vi "Multiscale Pyramids.vi"() -> ()   [LabVIEW 2023]
uses:
  Images/_Images.ctl
  SubVIs/FLT/Conv Flt Presets.ctl
  <vilib>/vision/NI_Vision_Development_Module.lvlib
panel:
  out "Pyr Levels":i32=9
  in  "Filters":T1[](array[typedef])=[enum."Seifert 7x7", enum."Seifert 5x5", enum."Highlight Details 3x3", enum."None", enum."None", enum."None", enum."None", enum."None", enum."None", enum."None", enum."None", enum."None"]
  out "Histogram":T2(graph)
  in  "Operator":u16(ring)=6 items=["Linear", "Log", "Exp", "Square", "Square root", "Power X", "Power 1/X"]
  in  "X Value":sgl=1.2 format="%.2f"
  in  "Threshold":sgl=30.0
  in  "Radius":sgl=33.0
  in  "Amount":sgl=6.0
  in  "LUT Multiplier":sgl[](array[slide])=[157.53847, 185.1077, 192.98462, 248.12308, 196.92308, 248.12308, 252.06154, 114.215385, 248.12308, 110.276924, 102.4, 102.4] scale=0.0..512.0
  in  "LUT Power":sgl[](array[slide])=[0.61538464, 0.43076923, 0.3846154, 0.43846154, 0.42307693, 0.5538462, 0.64615387, 0.61538464, 0.61538464, 0.6, 0.4, 0.4] scale=0.0..2.0
  out "Reconstructed Image":T3(plugin-control)
  out "Source Image":T3(plugin-control)
  in  "Image":T4=enum."Part1"
  # "Multoscale Contrast Enhancement using Pyramids"
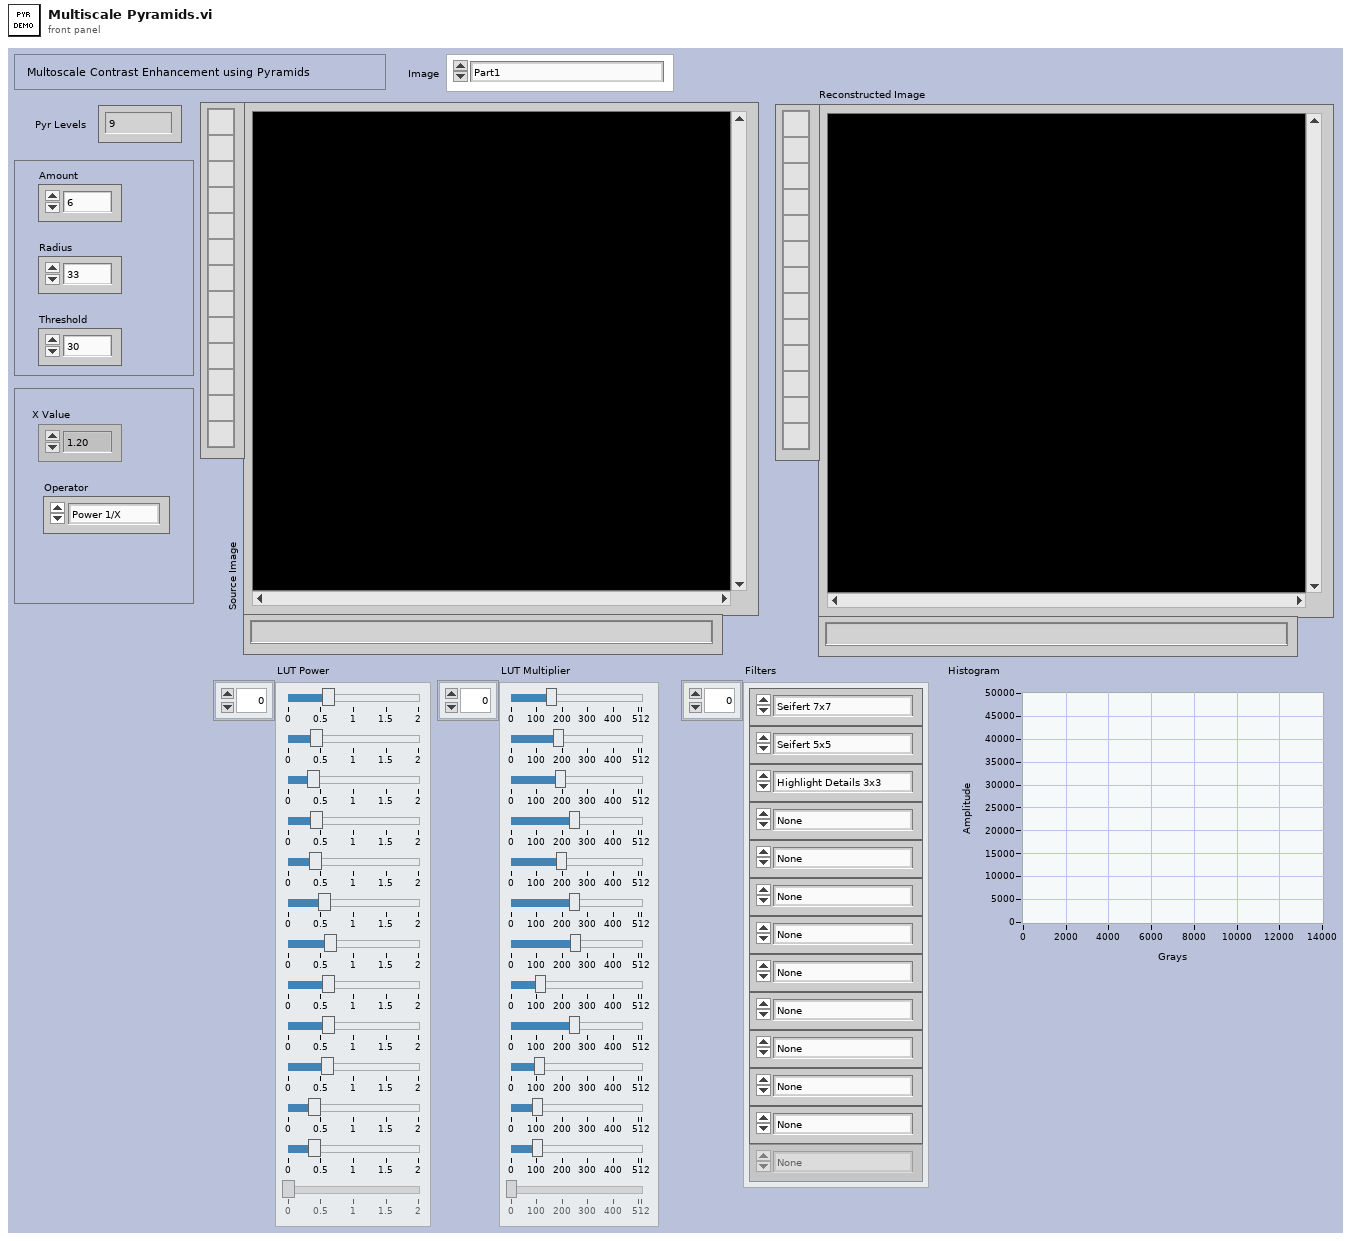
[diagram p1: front panel]
types:
  T1 = typedef "Conv Flt Presets.ctl" = enum16{"None", "Seifert 5x5", "Seifert 7x7", "High Pass 5x5 ", "High Pass 7x7", "Highlight Details 3x3", "Highlight Details 5x5", "Highlight Detail 7x7"}
  T2 = cluster{"Starting Value":sgl, "Incremental Value":sgl, "Histogram":u32[]}
  T3 = typedef "IMAQ Image.ctl" = refnum<image>
  T4 = typedef "_Images.ctl" = enum16{"Balls2", "Battery1", "Battery2", "Connector1", "Subwoofer1", "Subwoofer2", "Subwoofer3", "Subwoofer4", "Hase1", "Lamp1", "Lamp2", "Mouse1", "PhotoLens1", "Po1", "PowerSupply1", "Router", "--- Step Wedges ---", "Stepwedge1", "Stepwedge2", "Stepwedge3", "--- Fusion ---", "Fusion160kV", "Fusion2-120kV", "Fusion2-320kV", "Fusion300kV", "FusionPart1-120kV", "FusionPart1-180kV", "--- PART 01 ---", "Part1", "Part2", "Part3", "Part4", "Part5", "Part6", "Part7", "Part8", "--- Different Integrations ---", "Step2737-02Int", "Step2737-04Int", "Step2737-08Int", "Step2737-16Int", "Step2737-32Int", "Step2737-64Int"}
  T5 = typedef "Image Type" = u32
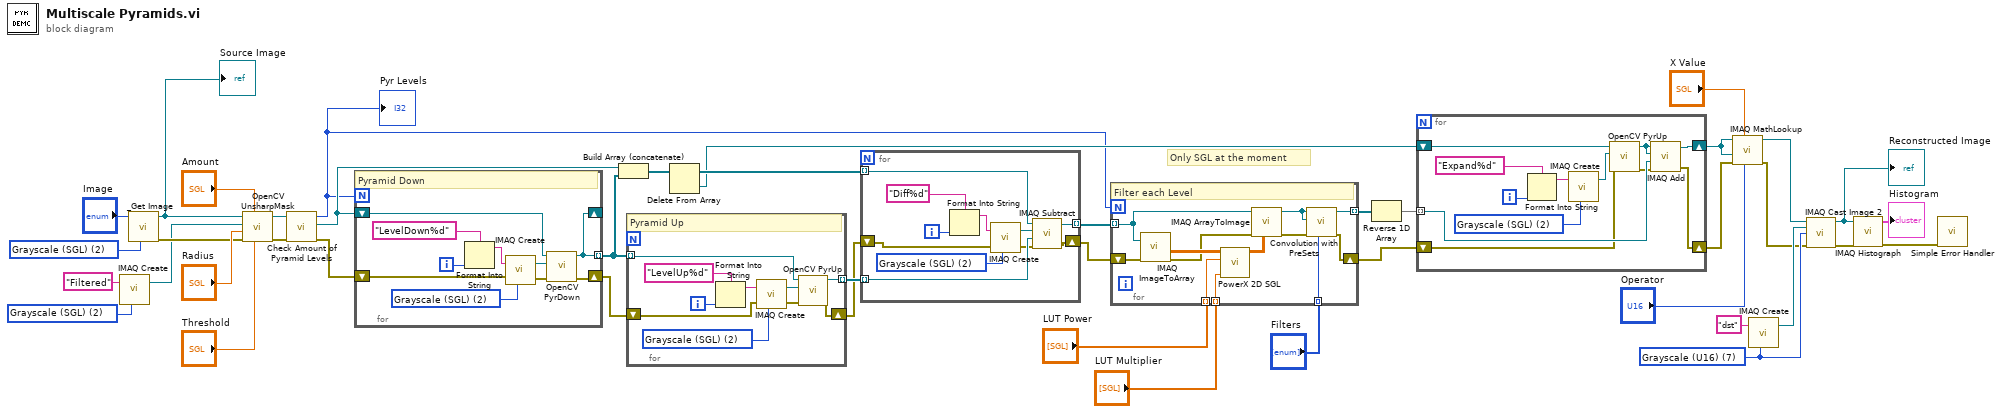
[diagram p0: block diagram]
diagram:
  w8 = T5 2 items=["Grayscale (U8)", "Grayscale (I16)", "Grayscale (SGL)", "Complex (CSG)", "RGB (U32)", "HSL (U32)", "RGB (U64)", "Grayscale (U16)"] ("Image Type")
  w34 = T5 7 items=["Grayscale (U8)", "Grayscale (I16)", "Grayscale (SGL)", "Complex (CSG)", "RGB (U32)", "HSL (U32)", "RGB (U64)", "Grayscale (U16)"] ("Image Type")
  w33 = T5 2 items=["Grayscale (U8)", "Grayscale (I16)", "Grayscale (SGL)", "Complex (CSG)", "RGB (U32)", "HSL (U32)", "RGB (U64)", "Grayscale (U16)"] ("Image Type (U16)")
  # "Only SGL at the moment"
  n1 = call "IMAQ Create"("Image Name"="Filtered", "Image Type"=w8) -> ("New Image"=w7:T3)  [unwired: 3 in, 1 out]
  n2 = call "_Get Image.vi"("Image Type (U16)"=w33, "Image"="Image") -> ("error out"=w20:errorcluster, "Image Out"=w1:T3)  [unwired: 6 in, 2 out]
  "Source Image" <- w1
  n3 = call "OpenCV UnsharpMask.vi"("Threshold"="Threshold", "Amount"="Amount", "error in (no error)"=w20, "Radius"="Radius", "Image Dst"=w7, "Image Src"=w1) -> ("error out"=w11:errorcluster, "Image Dst Out"=w6:T3)  [unwired: 4 in]
  n4 = call "Check Amount of Pyramid Levels.vi"("error in (no error)"=w11, "Refnum in"=w6) -> ("error out"=w10:errorcluster, "Image Dup"=w5:T3, "Pyr Levels"=w4:i32)  [unwired: 7 in]
  "Pyr Levels" <- w4
  n5 = for {
    N: w4 -> [_]
    shift-right: [w48] -> _
    shift-left: w5 -> [w50]
    tunnel: [w48] -> w22 mode=indexing
    shift-right: [w44] -> w19
    shift-left: w10 -> [w46]
    i -> [w47]
    w52 = T5 2 items=["Grayscale (U8)", "Grayscale (I16)", "Grayscale (SGL)", "Complex (CSG)", "RGB (U32)", "HSL (U32)", "RGB (U64)", "Grayscale (U16)"] ("Image Type")
    # "Pyramid Down"
    n6 = Format Into String(format string="LevelDown%d", w47) -> (resulting string=w51:string)  [unwired: 2 in, 1 out]
    n7 = call "IMAQ Create"("Image Name"=w51, "Image Type"=w52, "error in (no error)"=w46) -> ("New Image"=w49:T3, "error out"=w45:errorcluster)  [unwired: 2 in]
    n8 = call "OpenCV PyrDown.vi"("error in (no error)"=w45, "Image Dst"=w49, "Image Src"=w50) -> ("error out"=w44:errorcluster, "Image Dst Out"=w48:T3)  [unwired: 7 in]
  }
  n9 = Build Array (concatenate)(w5, w22) -> (w42:T3[])
  n10 = for {
    tunnel: [w59] -> w40 mode=indexing
    tunnel: w22 -> [w58] mode=indexing
    shift-right: [w54] -> w18
    shift-left: w19 -> [w56]
    i -> [w57]
    w62 = T5 2 items=["Grayscale (U8)", "Grayscale (I16)", "Grayscale (SGL)", "Complex (CSG)", "RGB (U32)", "HSL (U32)", "RGB (U64)", "Grayscale (U16)"] ("Image Type")
    # "Pyramid Up"
    n11 = Format Into String(format string="LevelUp%d", w57) -> (resulting string=w61:string)  [unwired: 2 in, 1 out]
    n12 = call "IMAQ Create"("Image Name"=w61, "Image Type"=w62, "error in (no error)"=w56) -> ("New Image"=w60:T3, "error out"=w55:errorcluster)  [unwired: 2 in]
    n13 = call "OpenCV PyrUp.vi"("error in (no error)"=w55, "Image Dst"=w60, "Image Src"=w58) -> ("error out"=w54:errorcluster, "Image Dst Out"=w59:T3)  [unwired: 7 in]
  }
  n14 = Delete From Array(array=w42) -> (deleted portion=w39:T3, array with subset deleted=w41:T3[])  [unwired: 2 in]
  n15 = for {
    tunnel: w41 -> [w70] mode=indexing
    tunnel: w40 -> [w69] mode=indexing
    tunnel: [w67] -> w30 mode=indexing
    shift-right: [w64] -> w17
    shift-left: w18 -> [w66]
    i -> [w71]
    w73 = T5 2 items=["Grayscale (U8)", "Grayscale (I16)", "Grayscale (SGL)", "Complex (CSG)", "RGB (U32)", "HSL (U32)", "RGB (U64)", "Grayscale (U16)"] ("Image Type")
    n16 = Format Into String(format string="Diff%d", w71) -> (resulting string=w74:string)  [unwired: 2 in, 1 out]
    n17 = call "IMAQ Create"("Image Name"=w74, "Image Type"=w73, "error in (no error)"=w66) -> ("New Image"=w68:T3, "error out"=w65:errorcluster)  [unwired: 2 in]
    n18 = call "IMAQ Subtract"("Image Src A"=w70, "Image Dst"=w68, "Image Src B"=w69, "error in (no error)"=w65) -> ("Image Dst Out"=w67:T3, "error out"=w64:errorcluster)  [unwired: 3 in]
  }
  n19 = for {
    N: w4 -> [_]
    tunnel: w30 -> [w86] mode=indexing
    tunnel: [w85] -> w37 mode=indexing
    tunnel: "LUT Power" -> [w81] mode=indexing
    tunnel: "LUT Multiplier" -> [w80] mode=indexing
    tunnel: "Filters" -> [w79] mode=indexing
    shift-right: [w75] -> w16
    shift-left: w17 -> [w76]
    # "Filter each Level"
    n20 = call "IMAQ ImageToArray"("error in (no error)"=w76, "Image"=w86) -> ("Image Pixels (Float)"=w83:sgl[][], "error out"=w78:errorcluster)  [unwired: 2 in, 3 out]
    n21 = call "PowerX 2D SGL.vi"("Multiplier"=w80, "Power"=w81, "Signal In"=w83) -> ("Signal Out"=w82:sgl[][])  [unwired: 8 in]
    n22 = call "IMAQ ArrayToImage"("Image Pixels (Float)"=w82, "error in (no error)"=w78, "Image"=w86) -> ("error out"=w77:errorcluster, "Image Out"=w84:T3)  [unwired: 7 in]
    n23 = call "Convolution with PreSets.vi"("Filter"=w79, "error in (no error)"=w77, "Image Dst"=w84, "Image Src"=w84) -> ("error out"=w75:errorcluster, "Image Dst Out"=w85:T3)  [unwired: 5 in, 1 out]
  }
  n24 = Reverse 1D Array(array=w37) -> (reversed array=w38:T3[])
  n25 = for {
    shift-right: [w90] -> w28
    shift-left: w39 -> [w93]
    tunnel: w38 -> [w91] mode=indexing
    shift-right: [w87] -> w15
    shift-left: w16 -> [w89]
    i -> [w94]
    w97 = T5 2 items=["Grayscale (U8)", "Grayscale (I16)", "Grayscale (SGL)", "Complex (CSG)", "RGB (U32)", "HSL (U32)", "RGB (U64)", "Grayscale (U16)"] ("Image Type")
    n26 = Format Into String(format string="Expand%d", w94) -> (resulting string=w96:string)  [unwired: 2 in, 1 out]
    n27 = call "IMAQ Create"("Image Name"=w96, "Image Type"=w97) -> ("New Image"=w95:T3)  [unwired: 3 in, 1 out]
    n28 = call "OpenCV PyrUp.vi"("error in (no error)"=w89, "Image Dst"=w95, "Image Src"=w93) -> ("error out"=w88:errorcluster, "Image Dst Out"=w92:T3)  [unwired: 7 in]
    n29 = call "IMAQ Add"("Image Src A"=w92, "Image Dst"=w92, "Image Src B"=w91, "error in (no error)"=w88) -> ("Image Dst Out"=w90:T3, "error out"=w87:errorcluster)  [unwired: 3 in]
  }
  n30 = call "IMAQ MathLookup"("Operator"="Operator", "X Value"="X Value", "error in (no error)"=w15, "Image Dst"=w28, "Image Src"=w28) -> ("error out"=w14:errorcluster, "Image Dst Out"=w3:T3)  [unwired: 5 in]
  n31 = call "IMAQ Create"("Image Name"="dst", "Image Type"=w34) -> ("New Image"=w35:T3)  [unwired: 3 in, 1 out]
  n32 = call "IMAQ Cast Image 2"("Image Src"=w3, "Image Dst"=w35, "Image Type"=w34, "error in (no error)"=w14) -> ("Image Dst Out"=w2:T3, "error out"=w13:errorcluster)  [unwired: 10 in]
  "Reconstructed Image" <- w2
  n33 = call "IMAQ Histograph"("error in (no error)"=w13, "Image"=w2) -> ("error out"=w12:errorcluster, "Histogram Graph"=→"Histogram":T2)  [unwired: 6 in, 2 out]
  n34 = call <vilib>:"Simple Error Handler.vi"("error in (no error)"=w12) -> ()  [unwired: 4 in, 5 out]
